vi "RT-HS-Parallel-Port.vi"() -> ()   [LabVIEW 2016]
uses:
  <vilib>/rvi/interface/nirviOpenFPGA/nirviOpenFPGA.xnode
  <vilib>/rvi/interface/nirviMethod/nirviMethod.xnode
  <vilib>/rvi/errors/niLvFpgaMergeErrorWithErrorCode.vi
  <vilib>/FPGAPlugInAG/Dynamic/niLvFpga_AcknowledgeIrq_Dynamic.vi
  <vilib>/rvi/interface/nirviMethod/StockFPGA_InlinedMethodWaitForSingleIRQ.vi
  <vilib>/FPGAPlugInAG/Dynamic/niLvFpga_WaitOnIrq_Dynamic.vi
  <vilib>/FPGAPlugInAG/Dynamic/niLvFpga_ConfigureFifo_Dynamic.vi
  <vilib>/FPGAPlugInAG/Dynamic/niLvFpga_ReadFifo_Dynamic.vi
  <vilib>/rvi/interface/nirviCloseFPGA/nirviCloseFPGA.xnode
  <vilib>/FPGAPlugInAG/Dynamic/niLvFpga_Close_Dynamic.vi
  FPGA Bitfiles/MyRIO-HS-Paralle_FPGATarget_FPGA-HS-Parallel_x9ODx5NBTEA.lvbitx
  FPGA-HS-Parallel-Port-Receiver.vi
  <vilib>/FPGAPlugInAG/myRIO-1900/niLvFpga_Open_myRIO-1900.vi
  <vilib>/rvi/interface/common/dynamic/niFpgaDynamicAddResources.vi
  <vilib>/NI/STM/NI STM.lvlib
  <vilib>/NI/STM/TCP/Write Meta Data (TCP Ref).vi
  <vilib>/NI/STM/SubVIs/MetaDataElement.ctl
panel:
  out "Actual Depth":u32
  out "Data":u32[](array[numeric])
  out "error out":errorcluster
  in  "Timeout (ms)":i32=5000
  in  "#Samples":u32
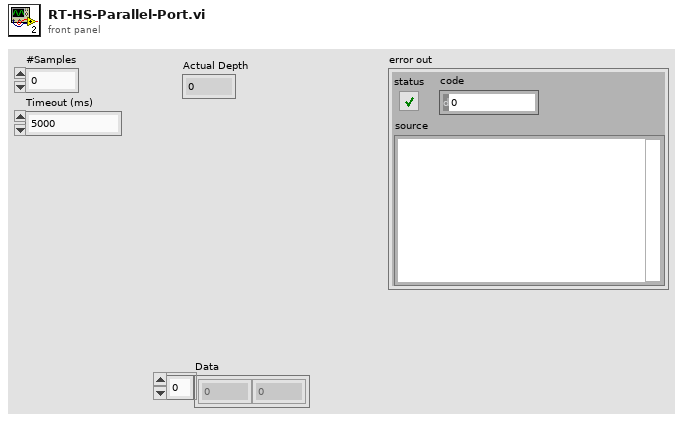
[diagram p1: front panel]
types:
  T1 = typedef "NI STM.lvlib/MetaDataElement.ctl" = string
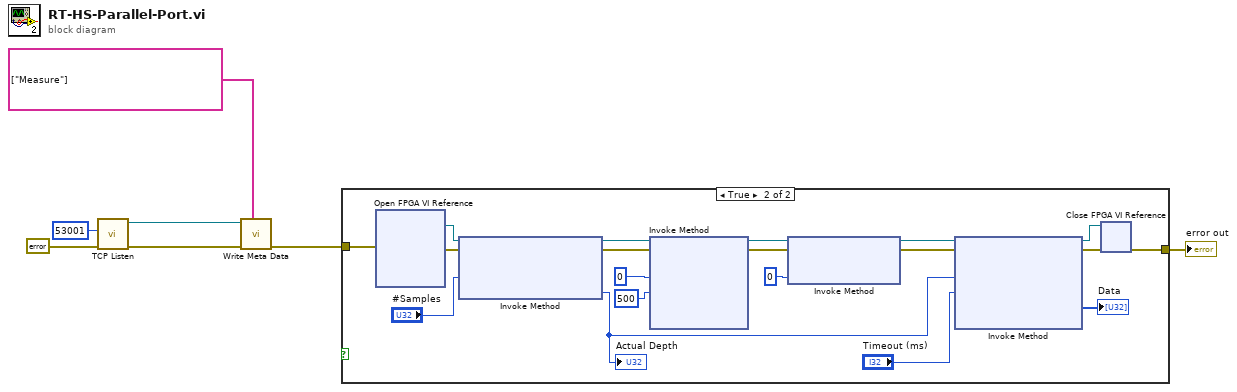
[diagram p0: block diagram]
diagram:
  n1 = call <vilib>:"TCP Listen.vi"("error in (no error)"=errorcluster {"status"=FALSE, "code"=0, "source"=""}, "port"=u16 53001) -> ("error out"=w5:errorcluster, "connection ID"=w6:refnum<k5>)  [unwired: 5 in, 3 out]
  n2 = call-poly <vilib>:"Write Meta Data.vi"("meta data"=T1[] ["Measure"], "error in"=w5, "connection ID"=w6) -> ("error out"=w4:errorcluster)  [unwired: 7 in, 1 out]
  n3 = case shown="True" {
    selector: _ -> [_ _]
    tunnel: [_ w10] -> w7
    tunnel: w4 -> [_ w8]
    frame False {
    }
    frame True {
      n4 = xnode "Open FPGA VI Reference"("error in"=w8) -> ("FPGA VI Reference Out"=w26:refnum<k20>, "error out"=w25:errorcluster)  [unwired: 1 in]
      n5 = xnode "Invoke Method"("FPGA VI Reference In"=w26, "error in"=w25, "Requested Depth"="#Samples") -> ("FPGA VI Reference Out"=w20:refnum<k20>, "error out"=w19:errorcluster, "Actual Depth"=w13:u32)
      "Actual Depth" <- w13
      n6 = xnode "Invoke Method"("FPGA VI Reference In"=w20, "error in"=w19, "IRQ Number(s)"=0, "Timeout (ms)"=500) -> ("FPGA VI Reference Out"=w18:refnum<k20>, "error out"=w17:errorcluster)  [unwired: 2 out]
      n7 = xnode "Invoke Method"("FPGA VI Reference In"=w18, "error in"=w17, "IRQ Number(s)"=0) -> ("FPGA VI Reference Out"=w16:refnum<k20>, "error out"=w15:errorcluster)
      n8 = xnode "Invoke Method"("FPGA VI Reference In"=w16, "error in"=w15, "Number of Elements"=w13, "Timeout (ms)"="Timeout (ms)") -> ("FPGA VI Reference Out"=w12:refnum<k20>, "error out"=w11:errorcluster, "Data"=→"Data":u32[])  [unwired: 1 out]
      n9 = xnode "Close FPGA VI Reference"("FPGA VI Reference In"=w12, "error in"=w11) -> ("error out"=w10:errorcluster)
    }
  }
  "error out" <- w7
